vi "setStopServerOcc.vi"(8 "error in (no error)":errorcluster, 11 "TcpServerBase in":refnum<class "TcpServerBase.lvclass">) -> (0 "error out":errorcluster, 3 "TcpServerBase out":refnum<class "TcpServerBase.lvclass">)   [LabVIEW 2018, in "TcpServerBase.lvclass"]
doc: "Set the stopServer occurrence to stop the servers."
uses:
  TcpServerBase.lvclass
  TcpServerBase.lvclass/TcpServerBase.ctl
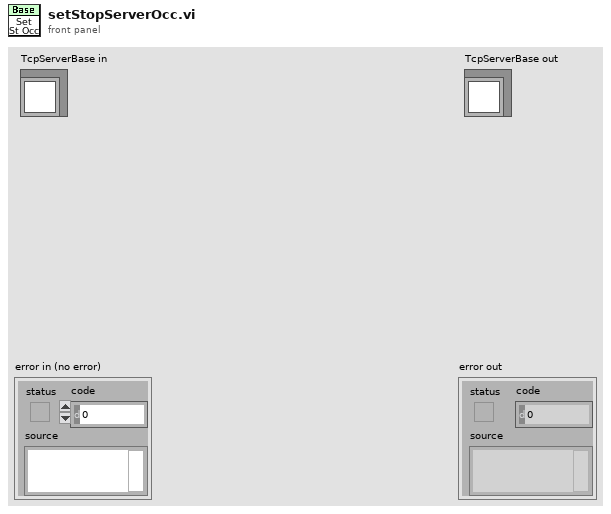
[diagram p1: front panel]
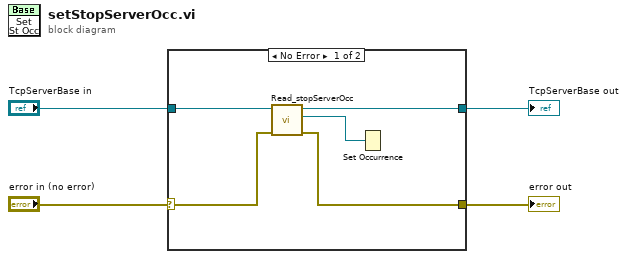
[diagram p0: block diagram]
diagram:
  n1 = case shown="No Error" "error in (no error)" {
    selector: "error in (no error)" -> [w6 w11]
    tunnel: [w5 w11] -> w3
    tunnel: [w7 w10] -> w1
    tunnel: "TcpServerBase in" -> [w8 w10]
    frame No Error {
      n2 = call "Read_stopServerOcc.vi"("error in (no error)"=w6, "TcpServerBase in"=w8) -> ("error out"=w5:errorcluster, "stopServerOcc"=w9:refnum<k4>, "TcpServerBase out"=w7:refnum<class "TcpServerBase.lvclass">)  [unwired: 7 in]
      n3 = Set Occurrence(w9) -> ()
    }
    frame Error {
    }
  }
  "error out" <- w3
  "TcpServerBase out" <- w1
